vi "Add Project Tasks.vi"(8 "error in (no error)":errorcluster, 9 "Tasks":string[](array[string]), 10 "Project Name":string, 11 "Projects in":refnum<class "Projects.lvclass">) -> (0 "error out":errorcluster, 2 "Success?":bool, 3 "Projects out":refnum<class "Projects.lvclass">)   [LabVIEW 2020, in "Projects.lvclass"]
doc: "Adds the tasks listed in the Tasks array to the Set data for Tasks for the Project Name provided. No data will be added if the Project Name is empty or is not present in the Map data. The Success? indicator will return True the Tasks are added, otherwise it will return False.\n\nUpdate: 10/2025 Because of the change to the Project Info in the Project Map, added a check in the Active Map to add a Map item to the Tasks Active with the Active boolean set to True.\n\n03/2025 Erich Schlieper"
uses:
  Projects.lvclass
  Projects.lvclass/Projects.ctl
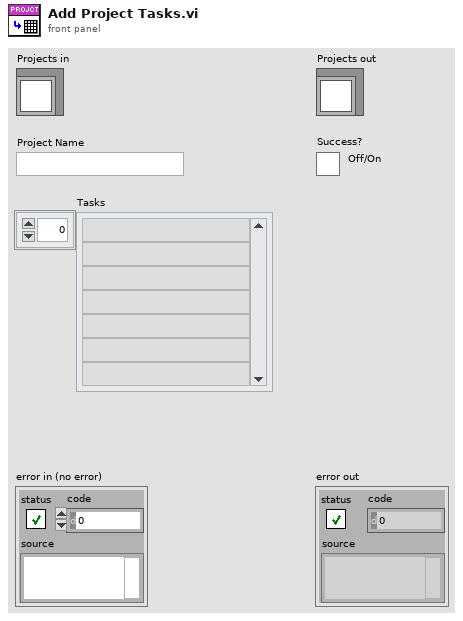
[diagram p1: front panel]
types:
  T1 = typedef "Project Info.ctl" = cluster{"Project Active?":bool, "Tasks":set{string}, "Task Active":map{string, bool}}
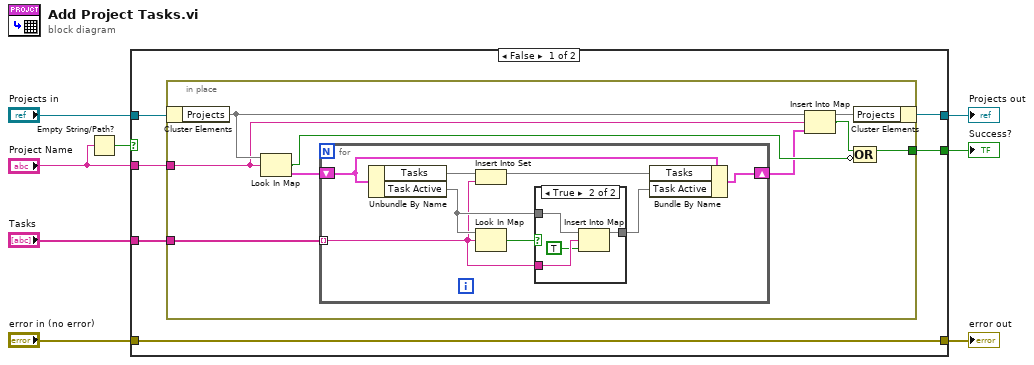
[diagram p0: block diagram]
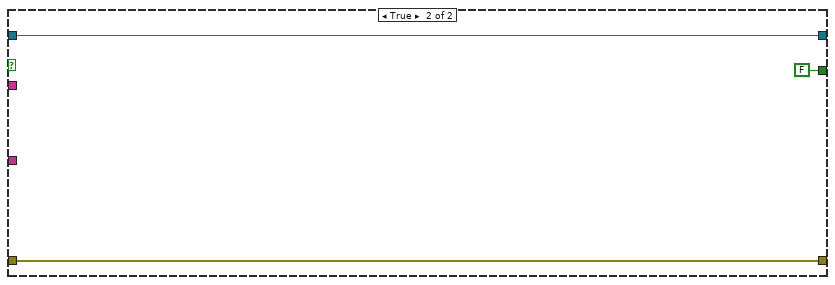
[diagram p3: hidden frame]
diagram:
  n1 = Empty String/Path?(string/path="Project Name") -> (empty?=w2:bool)
  n2 = case shown="False" w2 {
    tunnel: [w13 w39] -> w7
    tunnel: [w12 w38] -> w5
    tunnel: "Projects in" -> [w14 w38]
    tunnel: "Project Name" -> [w11 _]
    tunnel: "Tasks" -> [w10 _]
    tunnel: "error in (no error)" -> [w13 w39]
    tunnel: [w9 FALSE] -> w1
    frame False {
      n3 = in-place {
        in-place-border: w11 -> [w16]
        in-place-border: w10 -> [w23]
        in-place-border: [w18] -> w9
        n4 = in-place-cluster #1(w14) -> ("Projects"=w21:map{string, T1})
        n5 = Look In Map(map=w21, key=w16) -> (key not found?=w17:bool, value=w22:T1)  [unwired: 1 in]
        n6 = for {
          tunnel: w23 -> [w24] mode=indexing
          shift-right: [w29] -> w15
          shift-left: w22 -> [w28]
          n7 = Unbundle By Name(w28) -> ("Tasks"=w30:set{string}, "Task Active"=w26:map{string, bool})
          n8 = Insert Into Set(10:w24, 11:w30) -> (3:w31:set{string})  [unwired: 1 out]
          n9 = Look In Map(map=w26, key=w24) -> (key not found?=w27:bool)  [unwired: 1 in, 1 out]
          n10 = case shown="True" w27 {
            tunnel: w26 -> [w32 w36]
            tunnel: [w32 w35] -> w25
            tunnel: w24 -> [_ w34]
            frame False {
            }
            frame True {
              n11 = Insert Into Map(map in=w36, key=w34, value=TRUE) -> (map out=w35:map{string, bool})  [unwired: 2 out]
            }
          }
          n12 = Bundle By Name(cluster=w28, "Tasks"=w31, "Task Active"=w25) -> (w29:T1)
        }
        n13 = Insert Into Map(map in=w21, key=w16, value=w15) -> (map out=w20:map{string, T1}, key already included?=w19:bool)  [unwired: 1 out]
        n14 = in-place-cluster #1("Projects"=w20) -> (w12:refnum<class "Projects.lvclass">)
        n15 = Compound Arithmetic op=OR(w19, invert w17) -> (w18:bool)
      }
    }
    frame True {
    }
  }
  "error out" <- w7
  "Projects out" <- w5
  "Success?" <- w1
